vi "visa_test_2010sp1.vi"() -> ()   [LabVIEW 2010]
panel:
  out "error out":errorcluster
  in  "error in":errorcluster
  out "status 2":bool
  out "i 2":i32
  in  "stop 2":bool
  out "code 2":i32
  out "code":i32
  in  "stop":bool
  out "i":i32
  out "status":bool
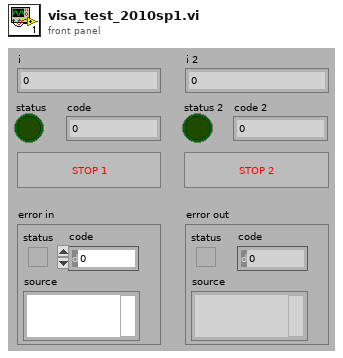
[diagram p1: front panel]
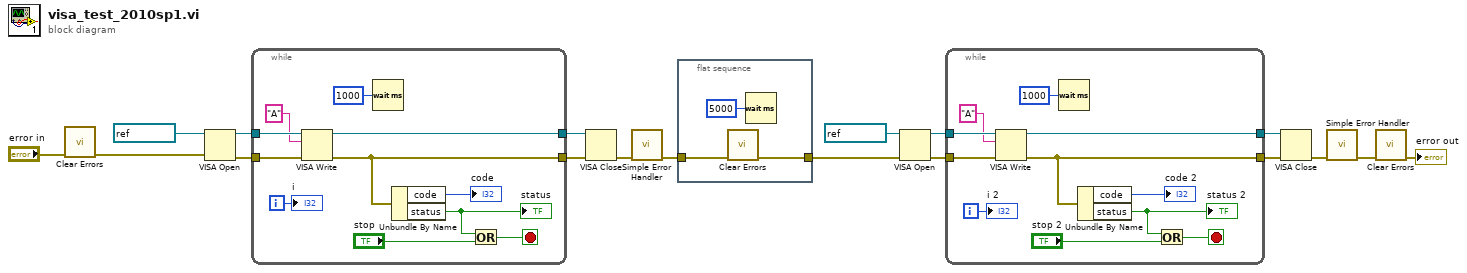
[diagram p0: block diagram]
diagram:
  n1 = call <vilib>:"Clear Errors.vi"("error in (no error)"="error in") -> ("error out"=w4:errorcluster)  [unwired: 6 in]
  n2 = VISA Open(error in (no error)=w4, VISA resource name=refnum<visa-resource-name> "COM3") -> (VISA resource name=w15:refnum<visa-resource-name>, error out=w17:errorcluster)  [unwired: 3 in]
  n3 = while {
    tunnel: [w24] -> w18
    tunnel: w17 -> [w25]
    tunnel: [w26] -> w16
    tunnel: w15 -> [w27]
    i -> [w28]
    stop <- w21 stop-if-true
    n4 = VISA Write(VISA resource name=w27, write buffer="A", error in (no error)=w25) -> (VISA resource name out=w26:refnum<visa-resource-name>, error out=w24:errorcluster)  [unwired: 1 out]
    n5 = Wait (ms)(milliseconds to wait=u32 1000) -> ()  [unwired: 1 out]
    n6 = Unbundle By Name(w24) -> ("code"=→"code":i32, "status"=w23:bool)
    "status" <- w23
    n7 = Or(x=w23, y="stop") -> (x .or. y?=w21:bool)
    "i" <- w28
  }
  n8 = VISA Close(VISA resource name=w16, error in (no error)=w18) -> (error out=w13:errorcluster)
  n9 = call <vilib>:"Simple Error Handler.vi"("error in (no error)"=w13) -> ("error out"=w12:errorcluster)  [unwired: 4 in, 4 out]
  n10 = flat-sequence {
    tunnel: w12 -> [w31]
    tunnel: [w30] -> w11
    frame #0 {
      n11 = call <vilib>:"Clear Errors.vi"("error in (no error)"=w31) -> ("error out"=w30:errorcluster)  [unwired: 6 in]
      n12 = Wait (ms)(milliseconds to wait=u32 5000) -> ()  [unwired: 1 out]
    }
  }
  n13 = VISA Open(error in (no error)=w11, VISA resource name=refnum<visa-resource-name> "COM3") -> (VISA resource name=w8:refnum<visa-resource-name>, error out=w9:errorcluster)  [unwired: 3 in]
  n14 = while {
    tunnel: [w38] -> w6
    tunnel: w9 -> [w39]
    tunnel: [w40] -> w5
    tunnel: w8 -> [w41]
    i -> [w42]
    stop <- w35 stop-if-true
    n15 = VISA Write(VISA resource name=w41, write buffer="A", error in (no error)=w39) -> (VISA resource name out=w40:refnum<visa-resource-name>, error out=w38:errorcluster)  [unwired: 1 out]
    n16 = Wait (ms)(milliseconds to wait=u32 1000) -> ()  [unwired: 1 out]
    n17 = Unbundle By Name(w38) -> ("code"=→"code 2":i32, "status"=w37:bool)
    "status 2" <- w37
    n18 = Or(x=w37, y="stop 2") -> (x .or. y?=w35:bool)
    "i 2" <- w42
  }
  n19 = VISA Close(VISA resource name=w5, error in (no error)=w6) -> (error out=w7:errorcluster)
  n20 = call <vilib>:"Simple Error Handler.vi"("error in (no error)"=w7) -> ("error out"=w2:errorcluster)  [unwired: 4 in, 4 out]
  n21 = call <vilib>:"Clear Errors.vi"("error in (no error)"=w2) -> ("error out"=→"error out":errorcluster)  [unwired: 6 in]
